vi "releaseNotifier.vi"(8 "error in (no error)":errorcluster, 11 "TcpServer in":refnum<class "TcpServer.lvclass">) -> (0 "error out":errorcluster, 3 "TcpServer out":refnum<class "TcpServer.lvclass">)   [LabVIEW 2018, in "TcpServer.lvclass"]
doc: "Release the stopServerProcessNotifier reference."
uses:
  TcpServer.lvclass
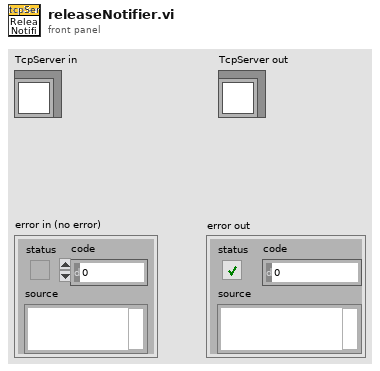
[diagram p1: front panel]
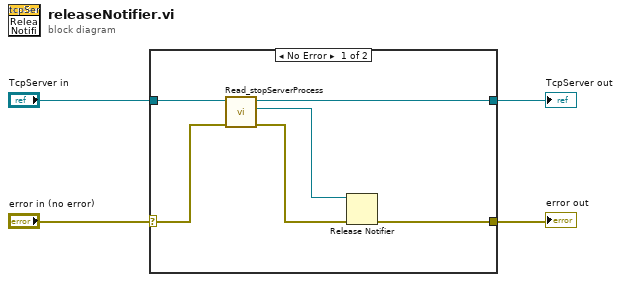
[diagram p0: block diagram]
diagram:
  n1 = case shown="No Error" "error in (no error)" {
    selector: "error in (no error)" -> [w9 w11]
    tunnel: "TcpServer in" -> [w7 w12]
    tunnel: [w6 w12] -> w2
    tunnel: [w5 w11] -> w1
    frame No Error {
      n2 = call-dynamic "Read_stopServerProcess.vi"("error in (no error)"=w9, "TcpServer in"=w7) -> ("error out"=w10:errorcluster, "stopServerProcessNotifier"=w8:refnum<notifier>, "TcpServer out"=w6:refnum<class "TcpServer.lvclass">)  [unwired: 7 in]
      n3 = Release Notifier(notifier=w8, error in (no error)=w10) -> (error out=w5:errorcluster)  [unwired: 1 in, 2 out]
    }
    frame Error {
    }
  }
  "TcpServer out" <- w2
  "error out" <- w1
